vi "PopSubpanel.vi"(8 "error in (no error)":errorcluster, 10 "Pop Index":i32, 11 "SMO.UI.MAUI in":refnum<class "SMO.UI.MAUI.lvclass">) -> (0 "error out":errorcluster, 3 "SMO.UI.MAUI out":refnum<class "SMO.UI.MAUI.lvclass">)   [LabVIEW 2016, in "SMO.UI.MAUI.lvclass"]
uses:
  SMO.UI.MAUI.lvclass
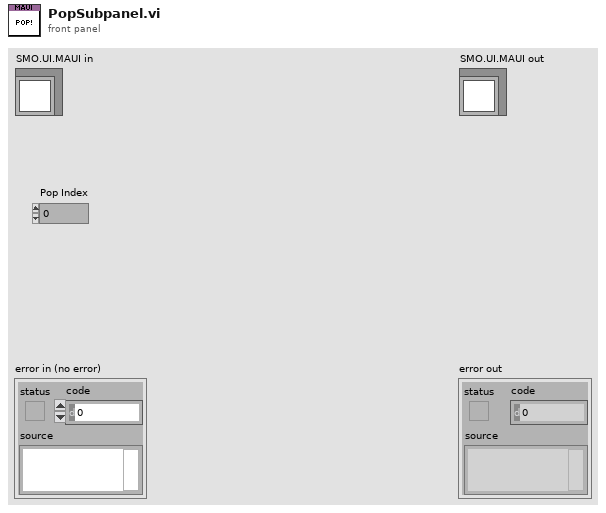
[diagram p1: front panel]
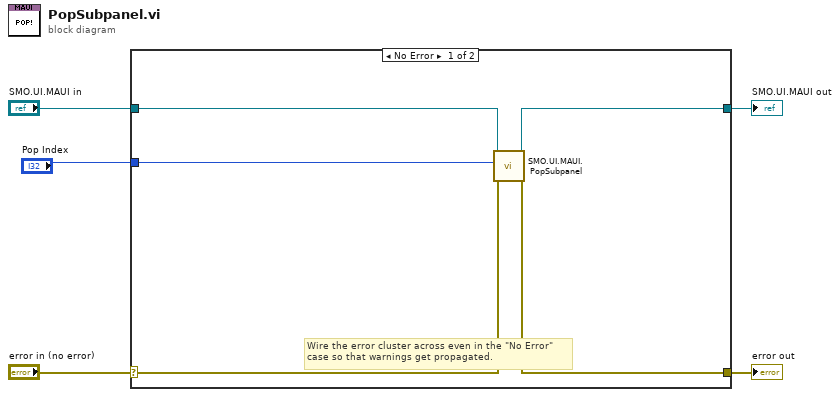
[diagram p0: block diagram]
diagram:
  n1 = case shown="No Error" "error in (no error)" {
    selector: "error in (no error)" -> [w9 w12]
    tunnel: [w8 w12] -> w4
    tunnel: [w6 w11] -> w2
    tunnel: "SMO.UI.MAUI in" -> [w7 w11]
    tunnel: "Pop Index" -> [w10 _]
    frame No Error {
      # "Wire the error cluster across even in the \"No Error\"\ncase so that warnings get propagated."
      n2 = call "SMO.UI.MAUI.PopSubpanel.vi"("error in (no error)"=w9, "PopSubpanel"=w10, "SMO.UI.MAUI"=w7) -> ("error out"=w8:errorcluster, "SMO.UI.MAUI out"=w6:refnum<class "SMO.UI.MAUI.lvclass">)  [unwired: 7 in]
    }
    frame Error {
    }
  }
  "error out" <- w4
  "SMO.UI.MAUI out" <- w2
